vi "E4_While_Loop.vi"() -> ()   [LabVIEW 2020]
panel:
  in  "STOP":bool
  out "Result1":i32
  out "Result4":i32
  out "Result3":i32
  out "Result2":i32
  out "Numeric":i32
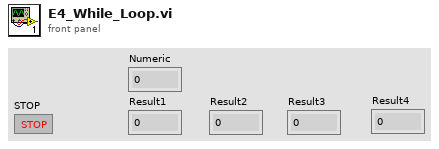
[diagram p1: front panel]
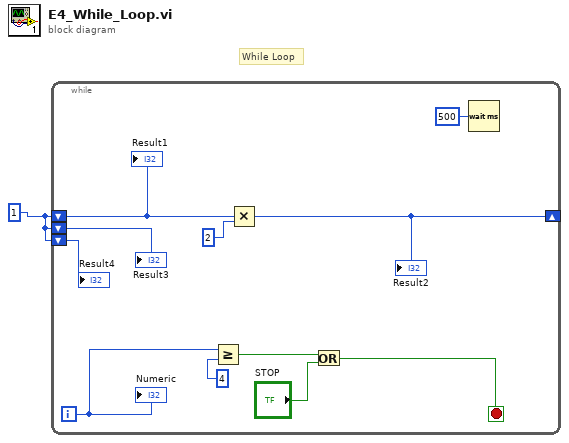
[diagram p0: block diagram]
diagram:
  w1 = 1
  # "While Loop"
  n1 = while {
    shift-right: [w9] -> _
    shift-left: w1 -> [w10]
    shift-left: w1 -> [w7]
    shift-left: w1 -> [w6]
    i -> [w5]
    stop <- w11 stop-if-true
    n2 = Greater Or Equal?(x=w5, y=4) -> (x >= y?=w4:bool)
    n3 = Multiply(x=w10, y=2) -> (x*y=w9:i32)
    "Result2" <- w9
    n4 = Or(x=w4, y="STOP") -> (x .or. y?=w11:bool)
    n5 = Wait (ms)(milliseconds to wait=u32 500) -> ()  [unwired: 1 out]
    "Numeric" <- w5
    "Result3" <- w7
    "Result4" <- w6
    "Result1" <- w10
  }
